vi "ALTS-2015 OPC Read LV2 Global.vi"(6 "OPC value Array":variant[](array[variant]), 7 "Options":T2, 8 "error in (no error)":errorcluster, 9 "OPC value":variant, 10 "OPC Read Register Array":T1[](array[typedef]), 11 "OPC Read Register":T1=enum."Start_Test") -> (0 "error out":errorcluster, 2 "OPC Read Register Array Value":variant[](array[variant]), 3 "OPC Read Reigter Value":variant)   [LabVIEW 2013]
uses:
  Controls/ALTS-2015 OPC Read Global Options.ctl
  Controls/ALTS-2015 OPC Read Registers.ctl
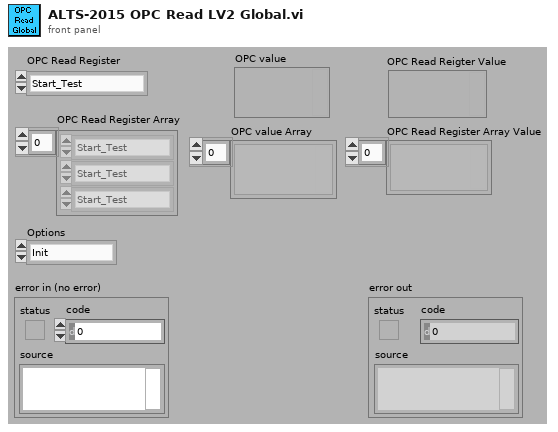
[diagram p1: front panel]
types:
  T1 = typedef "ALTS-2015 OPC Read Registers.ctl" = enum16{"Robot_Available", "Start_Test", "Stop_Test", "Scan_Trigger", "Station_No_Start_Stop_Test"}
  T2 = typedef "ALTS-2015 OPC Read Global Options.ctl" = enum16{"Init", "Write Value", "Write Array", "Read Value", "Read Array", "Read All"}
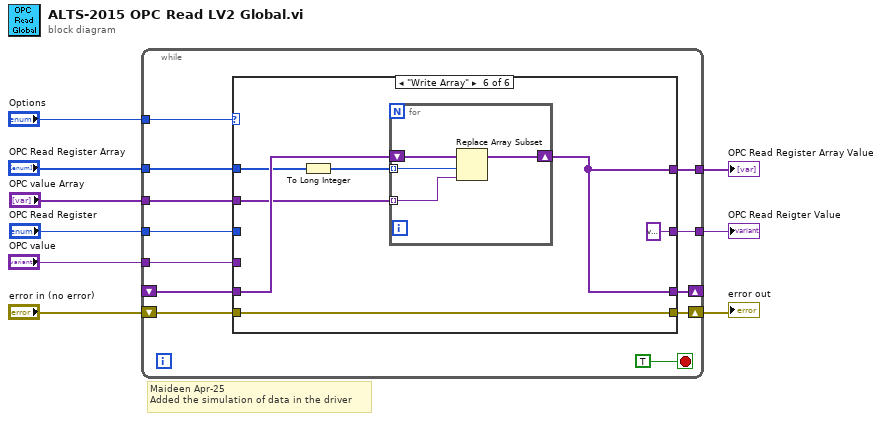
[diagram p0: block diagram]
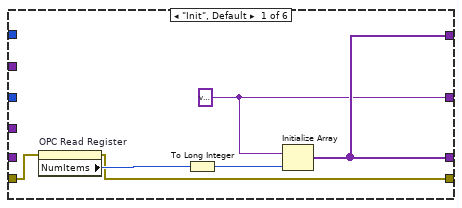
[diagram p2: hidden frame]
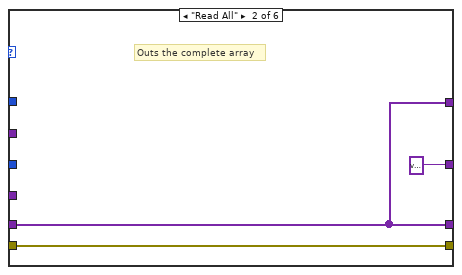
[diagram p3: hidden frame]
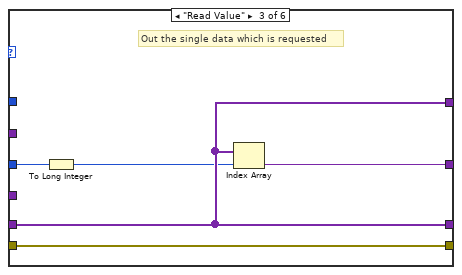
[diagram p4: hidden frame]
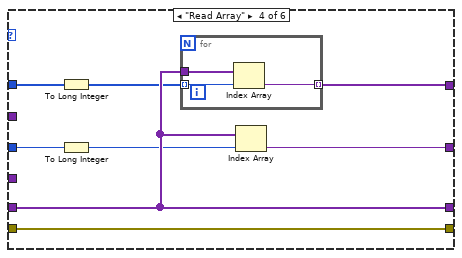
[diagram p5: hidden frame]
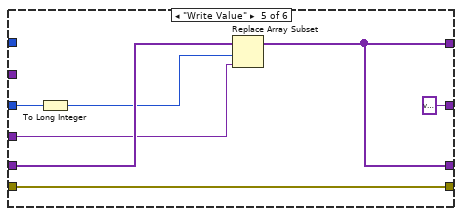
[diagram p6: hidden frame]
diagram:
  # "Maideen Apr-25\nAdded the simulation of data in the driver"
  n1 = while {
    shift-right: [w20] -> _
    shift-left: _ -> [w19]
    tunnel: "OPC Read Register Array" -> [w18]
    tunnel: "OPC Read Register" -> [w17]
    tunnel: [w16] -> w7
    tunnel: [w15] -> w6
    shift-right: [w13] -> w4
    shift-left: "error in (no error)" -> [w14]
    tunnel: "OPC value Array" -> [w12]
    tunnel: "OPC value" -> [w11]
    tunnel: "Options" -> [w10]
    stop <- TRUE stop-if-true
    n2 = case shown="\"Write Array\"" w10 {
      tunnel: [w27 w28 w33 w40 w53 w60] -> w20
      tunnel: w19 -> [_ w28 w33 w40 w51 w58]
      tunnel: w18 -> [_ _ _ w43 _ w56]
      tunnel: w17 -> [_ _ w35 w39 w49 _]
      tunnel: [w22 variant ("OPC value") w34 w38 variant ("OPC value") variant ("OPC value")] -> w16
      tunnel: [w27 w28 w33 w42 w53 w60] -> w15
      tunnel: w14 -> [w25 w30 w32 w41 w52 w59]
      tunnel: [w24 w30 w32 w41 w52 w59] -> w13
      tunnel: w12 -> [_ _ _ _ _ w57]
      tunnel: w11 -> [_ _ _ _ w50 _]
      frame "Init", Default {
        w22 = variant ("OPC value")
        n3 = property on="OPC Read Register" class="Enum (strict)"(error in=w25) -> (error out=w24:errorcluster, "NumItems"=w26:u32)  [unwired: 1 in, 1 out]
        n4 = To Long Integer(number=w26) -> (32bit integer=w23:i32)
        n5 = Initialize Array(w22, w23) -> (w27:variant[])
      }
      frame "Read All" {
        # "Outs the complete array"
      }
      frame "Read Value" {
        # "Out the single data which is requested"
        n6 = To Long Integer(number=w35) -> (32bit integer=w31:i32)
        n7 = Index Array(array=w33, index=w31) -> (element=w34:variant)
      }
      frame "Read Array" {
        n8 = To Long Integer(number=w43) -> (32bit integer=w36:i32[])
        n9 = To Long Integer(number=w39) -> (32bit integer=w37:i32)
        n10 = for {
          tunnel: w40 -> [w46]
          tunnel: w36 -> [w45] mode=indexing
          tunnel: [w44] -> w42 mode=indexing
          n11 = Index Array(array=w46, index=w45) -> (element=w44:variant)
        }
        n12 = Index Array(array=w40, index=w37) -> (element=w38:variant)
      }
      frame "Write Value" {
        n13 = To Long Integer(number=w49) -> (32bit integer=w48:i32)
        n14 = Replace Array Subset(array=w51, new element=w50, index=w48) -> (w53:variant[])
      }
      frame "Write Array" {
        n15 = To Long Integer(number=w56) -> (32bit integer=w55:i32[])
        n16 = for {
          tunnel: w57 -> [w62] mode=indexing
          shift-right: [w63] -> w60
          shift-left: w58 -> [w64]
          tunnel: w55 -> [w61] mode=indexing
          n17 = Replace Array Subset(array=w64, new element=w62, index=w61) -> (w63:variant[])
        }
      }
    }
  }
  "error out" <- w4
  "OPC Read Reigter Value" <- w7
  "OPC Read Register Array Value" <- w6
